vi "Periodic Tasks.vi"(8 "error in":errorcluster) -> ()   [LabVIEW 2014]
doc: "This VI runs in parallel to other tasks. It can contain as many user-defined periodic loops as you need. These can carry out PID or other sorts of timed response."
uses:
  <vilib>/Rock Robotics/Network Tables/SD Write String Array.vi
  Global Variables/Autonomous Play Globals.vi
  Global Variables/Miscalleneous.vi
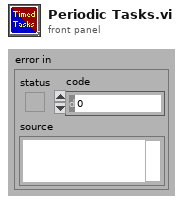
[diagram p1: front panel]
types:
  T1 = typedef "WPI_I2CDevRef.ctl" = cluster{"DevStatus":errorcluster, "Controller":T2, "Device Address":u8, "Handle":i32, "I2C Bus":T3}
  T2 = typedef "FPGA_TypedefDigitalModule.ctl" = enum16{"Controller 1"}
  T3 = typedef "i2c_bus.ctl" = enum16{"I2C On-Board", "I2C MXP", "Invalid"}
  T4 = typedef "Magnetometer Readings Cluster.ctl" = cluster{"X":i32, "Y":i32, "Z":i32}
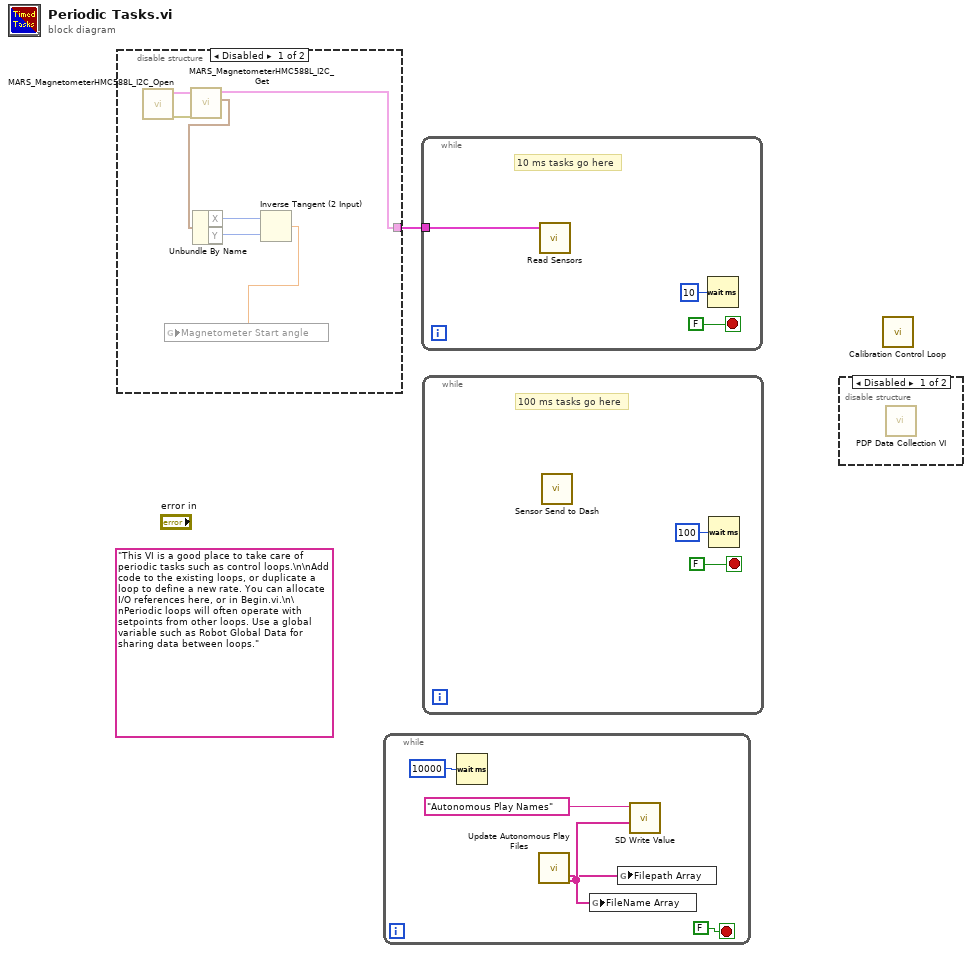
[diagram p0: block diagram]
diagram:
  (unwired) "This VI is a good place to take care of periodic tasks such as control loops.\n\nAdd code to the existing loops, or duplicate a loop to define a new rate. You can allocate I/O references here, or in Begin.vi.\n\nPeriodic loops will often operate with setpoints from other loops. Use a global variable such as Robot Global Data for sharing data between loops."
  n1 = disable-structure shown="Disabled" {
    disable-tunnel: [w6 _] -> w1
    frame Disabled {
      n2 = call "MARS_MagnetometerHMC588L_I2C_Open.vi"() -> ("error out"=w8:errorcluster, "I2CDevRef"=w7:T1)  [unwired: 10 in]
      n3 = call "MARS_MagnetometerHMC588L_I2C_Get.vi"("error in"=w8, "I2CDevRef"=w7) -> ("Magnetometer Reading"=w5:T4, "I2CDevRef 2"=w6:T1)  [unwired: 7 in, 1 out]
      n4 = Unbundle By Name(w5) -> ("X"=w4:i32, "Y"=w3:i32)
      n5 = Inverse Tangent (2 Input)(1:w3, 2:w4) -> (0:w2:dbl)
      n6 = global write "Miscalleneous.vi" "Magnetometer Start angle"(w2) -> ()
    }
    frame Enabled {
    }
  }
  n7 = while {
    stop <- FALSE stop-if-true
    n8 = Wait (ms)(milliseconds to wait=u32 10000) -> ()  [unwired: 1 out]
    n9 = call "Update Autonomous Play Files.vi"() -> ("Filepath Array"=w9:string[], "filename array"=w13:string[])  [unwired: 12 in, 2 out]
    n10 = global write "Autonomous Play Globals.vi" "FileName Array"(w13) -> ()
    n11 = global write "Autonomous Play Globals.vi" "Filepath Array"(w9) -> ()
    n12 = call-poly <vilib>:"SD Write Value.vi"("String Array"=w13, "Name"="Autonomous Play Names") -> ()  [unwired: 8 in, 2 out]
  }
  n13 = while {
    tunnel: w1 -> [w14]
    stop <- FALSE stop-if-true
    # "10 ms tasks go here"
    n14 = call "Read Sensors.vi"("MagnetometerRef"=w14) -> ()  [unwired: 11 in]
    n15 = Wait (ms)(milliseconds to wait=u32 10) -> ()  [unwired: 1 out]
  }
  n16 = while {
    stop <- FALSE stop-if-true
    # "100 ms tasks go here"
    n17 = call "Sensor Send to Dash.vi"() -> ()  [unwired: 12 in]
    n18 = Wait (ms)(milliseconds to wait=u32 100) -> ()  [unwired: 1 out]
  }
  n19 = disable-structure shown="Disabled" {
    frame Disabled {
      n20 = call "PDP Data Collection VI.vi"() -> ()  [unwired: 12 in]
    }
    frame Enabled {
    }
  }
  n21 = call "Calibration Control Loop.vi"() -> ()  [unwired: 12 in]
